vi "Launch Model.vi"(8 "error in (no error)":errorcluster, 11 "IController in":refnum<class "IController.lvclass">) -> (0 "error out":errorcluster, 3 "IController out":refnum<class "IController.lvclass">)   [LabVIEW 2015, in "IController.lvlib" / "IController.lvclass"]
uses:
  IController.lvclass
  IMediator/IMediator Messages/Publish Msg/Publish Msg.lvclass
  IController.lvclass/IController.ctl
  AbstractMessages/PreAddressedMsg/PreAddressedMsg.lvclass/PreAddressedMsg.ctl
  IModel/IModel/IModel.lvclass/IModel.ctl
  <vilib>/ActorFramework/Actor/Actor.lvclass
  IModel/IModel/IModel.lvclass
  AbstractMessages/PreAddressedMsg/PreAddressedMsg.lvclass
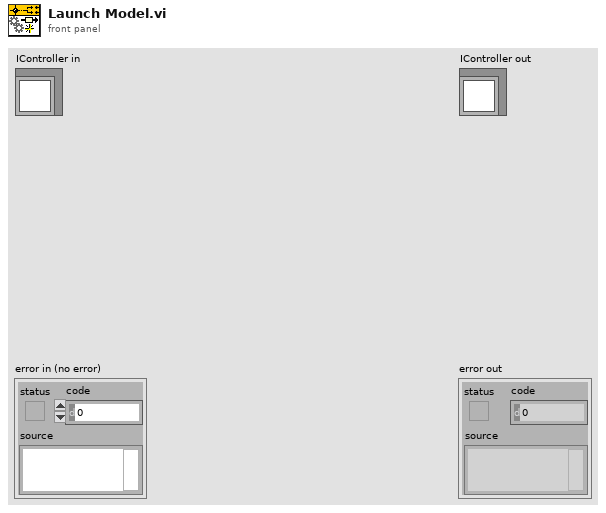
[diagram p1: front panel]
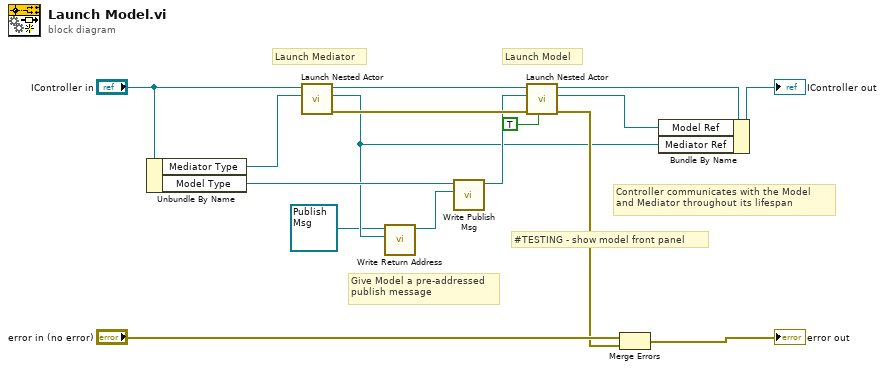
[diagram p0: block diagram]
diagram:
  # "#TESTING - show model front panel"
  # "Launch Model"
  # "Launch Mediator"
  # "Give Model a pre-addressed\npublish message"
  # "Controller communicates with the Model\nand Mediator throughout its lifespan"
  n1 = Unbundle By Name("IController in") -> ("Mediator Type"=w13:refnum<class "Mediator.lvclass">, "Model Type"=w12:refnum<class "IModel.lvclass">)
  n2 = call <vilib>:"Launch Nested Actor.vi"("Nested Actor"=w13, "Caller Actor in"="IController in") -> ("error out"=w8:errorcluster, "Nested Actor's Enqueuer"=w4:refnum<class "Message Enqueuer.lvclass">, "Caller Actor out"=w14:refnum<class "IController.lvclass">)  [unwired: 7 in]
  n3 = call "Write Return Address.vi"("Return Address"=w4, "PreAddressedMsg in"=refnum<class "Publish Msg.lvclass"> refnum ("IMediator.lvlib:Publish Msg.lvclass")) -> ("PreAddressedMsg out"=w3:refnum<class "Publish Msg.lvclass">)  [unwired: 9 in]
  n4 = call "Write Publish Msg.vi"("Pre-Addressed Publish Msg"=w3, "IModel in"=w12) -> ("IModel out"=w5:refnum<class "IModel.lvclass">)  [unwired: 9 in]
  n5 = call <vilib>:"Launch Nested Actor.vi"("Open Actor Core front panel? (F)"=TRUE, "error in (no error)"=w8, "Nested Actor"=w5, "Caller Actor in"=w14) -> ("error out"=w6:errorcluster, "Nested Actor's Enqueuer"=w9:refnum<class "Message Enqueuer.lvclass">, "Caller Actor out"=w11:refnum<class "IController.lvclass">)  [unwired: 5 in]
  n6 = Merge Errors("error in (no error)", w6) -> (→"error out":errorcluster)
  n7 = Bundle By Name(cluster=w11, "Model Ref"=w9, "Mediator Ref"=w4) -> (→"IController out":refnum<class "IController.lvclass">)
